vi "Find pulse in file.vi"(6 "Offset duration":dbl=0.1 format="%0.2f", 8 "Error In":errorcluster, 9 "Channel":string="CH0", 10 "group name in":string="Untitled", 11 "File Path Control":path) -> (0 "Error Out":errorcluster, 1 "duration":dbl=1.0 format="%0.2f", 2 "Start time":dbl, 3 "File Path out":path, 5 "Found":bool)   [LabVIEW 2015]
uses:
  <vilib>/measure/mamon.llb/Waveform Peak Detection for 1 Chan.vi
  <vilib>/Waveform/WDTOps.llb/WDT Get Waveform Subset DBL.vi
  <vilib>/measure/NI_MAPro.lvlib
panel:
  out "# peaks found":i32
  out "# valeys found":i32
  in  "Absolute noise floor":dbl=0.005 format="%#_6p"
  in  "Pad pulse":dbl=0.01 format="%#_6p"
  out "Peak Amplitudes":dbl[](array[numeric]) format="%.2p"
  out "Peak Locations":dbl[](array[numeric]) format="%.5p"
  out "Valley Amplitudes":dbl[](array[numeric]) format="%.2p"
  in  "Feature duration":dbl=8e-05 format="%#_6p"
  out "Valley Locations":dbl[](array[numeric]) format="%.5p"
  in  "Signal to noise ratio":dbl=40.0
  out "Y min":dbl format="%0.2f"
  out "Y max":dbl format="%0.2f"
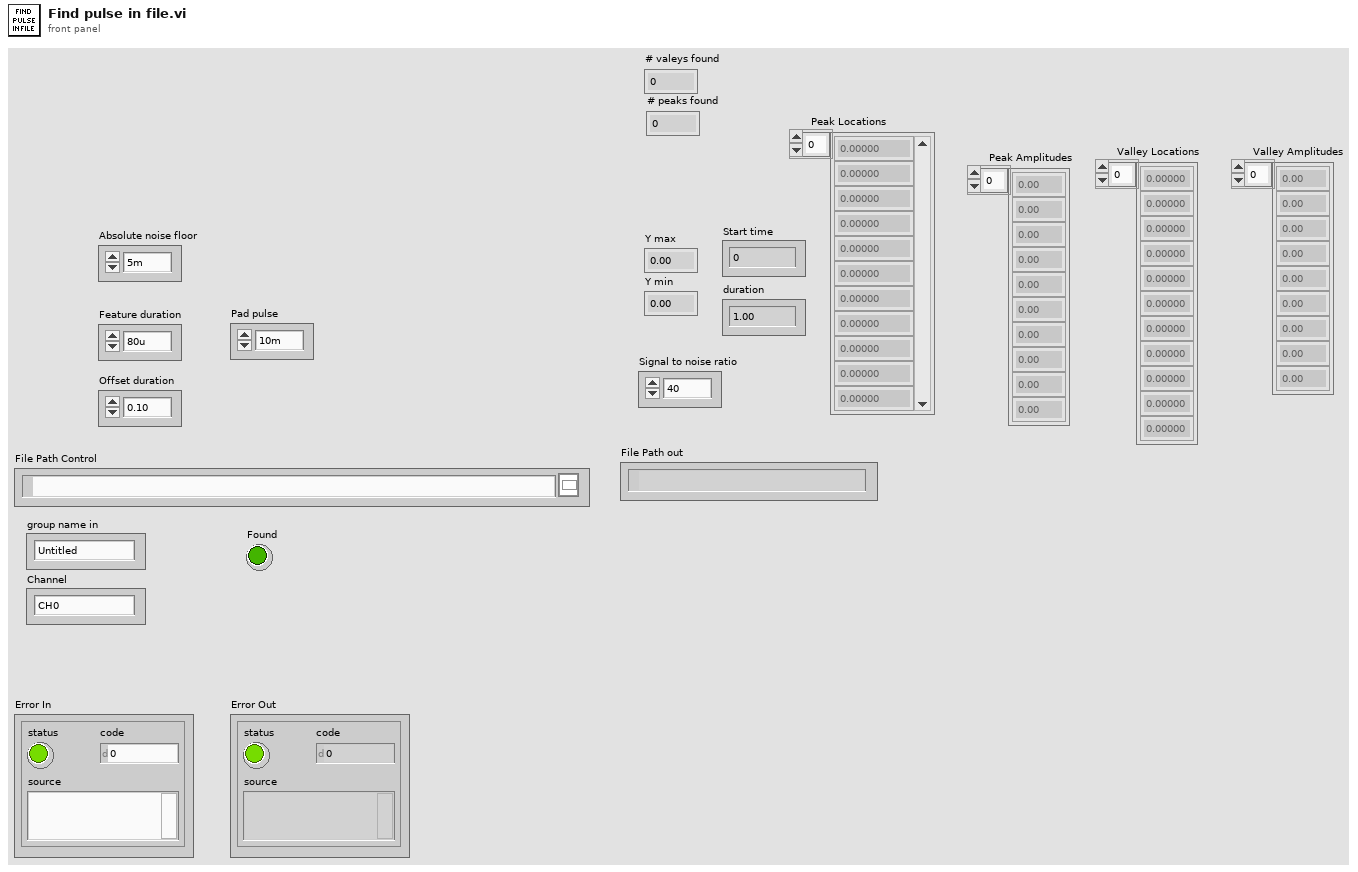
[diagram p1: front panel]
types:
  T1 = enum16{"open", "open or create", "create or replace", "create", "open (read-only)"}
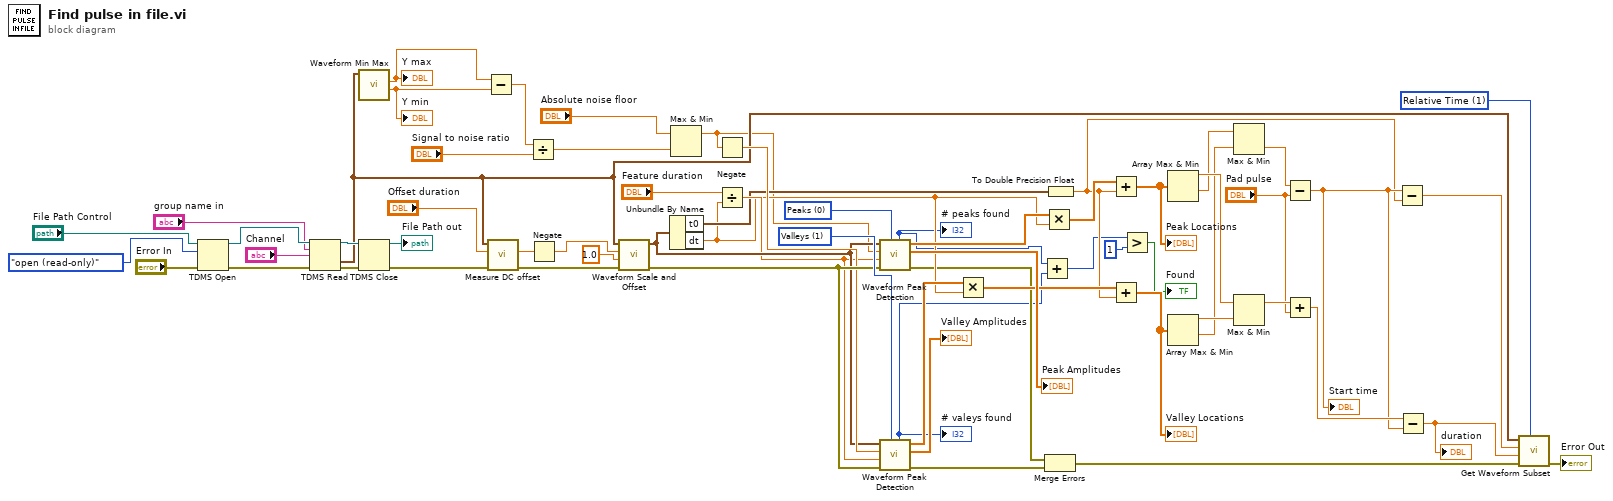
[diagram p0: block diagram]
diagram:
  w12 = u16 1 items=["Samples", "Relative Time"] ("start/duration format")
  w42 = u16 1 items=["Peaks", "Valleys"] ("peaks/valleys")
  w43 = u16 0 items=["Peaks", "Valleys"] ("peaks/valleys")
  n1 = TDMS Open(8:"Error In", 10:T1."open (read-only)" ("operation (0:open)"), 11:"File Path Control") -> (0:w61:errorcluster, 3:w62:refnum<k34>)  [unwired: 4 in]
  n2 = TDMS Read(0:w62, 5:"group name in", 7:"Channel", 11:w61) -> (4:w56:refnum<k34>, 10:w18:waveform(dbl), 15:w55:errorcluster)  [unwired: 4 in, 3 out]
  n3 = call <vilib>:"Waveform Min Max.vi"("waveform in"=w18) -> ("Y min"=w46:dbl, "Y max"=w47:dbl)  [unwired: 5 in, 4 out]
  "Y max" <- w47
  "Y min" <- w46
  n4 = TDMS Close(8:w55, 11:w56) -> (0:w53:errorcluster, 3:→"File Path out":path)
  n5 = Subtract(x=w47, y=w46) -> (x-y=w45:dbl)
  n6 = call "Measure DC offset.vi"("Error In"=w53, "Offset duration"="Offset duration", "Waveform"=w18) -> ("Error Out"=w50:errorcluster, "Offset"=w52:dbl)  [unwired: 7 in]
  n7 = Divide(x=w45, y="Signal to noise ratio") -> (x/y=w40:dbl)
  n8 = Negate(x=w52) -> (-x=w48:dbl)
  n9 = call <vilib>:"Waveform Scale and Offset.vi"("error in (no error)"=w50, "scale"=1.0, "offset"=w48, "waveform in"=w18) -> ("error out"=w41:errorcluster, "waveform out"=w36:waveform(dbl))  [unwired: 6 in]
  n10 = Unbundle By Name(w36) -> ("t0"=w33:timestamp, "dt"=w28:dbl)
  n11 = Max & Min(x="Absolute noise floor", y=w40) -> (max(x,y)=w7:dbl)  [unwired: 1 out]
  n12 = Negate(x=w7) -> (-x=w39:dbl)
  n13 = Divide(x="Feature duration", y=w28) -> (x/y=w34:dbl)
  n14 = call-poly <vilib>:"Waveform Peak Detection.vi"("peaks/valleys"=w43, "error in"=w41, "width"=w34, "threshold"=w7, "Signal In"=w36) -> ("error out"=w17:errorcluster, "Amplitudes"=→"Peak Amplitudes":dbl[], "Locations"=w32:dbl[], "# found"=w5:i32)  [unwired: 2 in, 1 out]
  "# peaks found" <- w5
  n15 = call-poly <vilib>:"Waveform Peak Detection.vi"("peaks/valleys"=w42, "error in"=w41, "width"=w34, "threshold"=w39, "Signal In"=w36) -> ("error out"=w16:errorcluster, "Amplitudes"=→"Valley Amplitudes":dbl[], "Locations"=w29:dbl[], "# found"=w4:i32)  [unwired: 2 in, 1 out]
  "# valeys found" <- w4
  n16 = Multiply(x=w29, y=w28) -> (x*y=w30:dbl[])
  n17 = Add(x=w5, y=w4) -> (x+y=w3:i32)
  n18 = Multiply(x=w32, y=w28) -> (x*y=w31:dbl[])
  n19 = Merge Errors(w17, w16) -> (w15:errorcluster)
  n20 = To Double Precision Float(number=w33) -> (double precision float=w10:dbl)
  n21 = Add(x=w31, y=w10) -> (x+y=w27:dbl[])
  "Peak Locations" <- w27
  n22 = Add(x=w30, y=w10) -> (x+y=w26:dbl[])
  "Valley Locations" <- w26
  n23 = Greater?(x=w3, y=1) -> (0:→"Found":bool)
  n24 = Array Max & Min(array=w27) -> (max value=w25:dbl, min value=w23:dbl)  [unwired: 2 out]
  n25 = Array Max & Min(array=w26) -> (max value=w24:dbl, min value=w22:dbl)  [unwired: 2 out]
  n26 = Max & Min(x=w23, y=w22) -> (min(x,y)=w20:dbl)  [unwired: 1 out]
  n27 = Max & Min(x=w25, y=w24) -> (max(x,y)=w21:dbl)  [unwired: 1 out]
  n28 = Subtract(x=w20, y="Pad pulse") -> (x-y=w11:dbl)
  "Start time" <- w11
  n29 = Add(x=w21, y="Pad pulse") -> (x+y=w14:dbl)
  n30 = Subtract(x=w11, y=w10) -> (x-y=w9:dbl)
  n31 = Subtract(x=w14, y=w11) -> (x-y=w6:dbl)
  "duration" <- w6
  n32 = call-poly <vilib>:"Get Waveform Subset.vi"("start/duration format"=w12, "error in (no error)"=w15, "duration"=w6, "start samples/time"=w9, "waveform in"=w18) -> ("error out"=→"Error Out":errorcluster)  [unwired: 1 in, 3 out]
